vi "Convert Class To Database.vi"(8 "error in (no error)":errorcluster, 10 "table":string, 11 "MemberInfo in":refnum<class "Information.lvclass">) -> (0 "error out":errorcluster, 2 "UserInfo":T1, 3 "MemberInfo out":refnum<class "Information.lvclass">)   [LabVIEW 2015, in "Member_Actor.lvlib" / "Information.lvclass"]
uses:
  Information.lvclass
  Type Definitions/UserInfo.ctl
  Information.lvclass/Information.ctl
  API/_Database/Database.lvclass
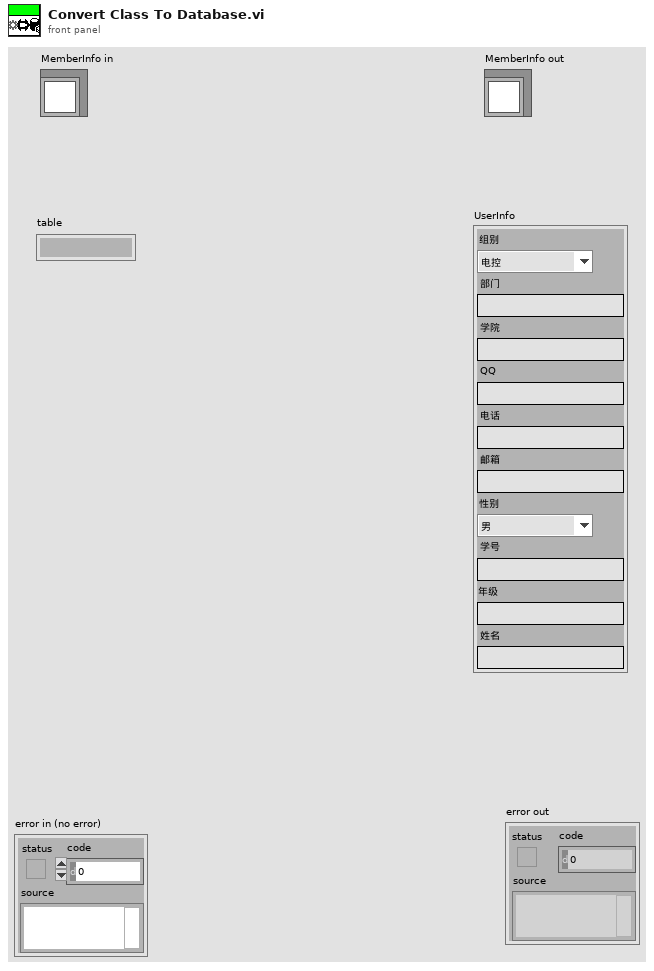
[diagram p1: front panel]
types:
  T1 = typedef "Member_Actor.lvlib/Information.lvclass/UserInfo.ctl" = cluster{"组别":enum16{"电控", "机械", "视觉"}, "部门":string, "学院":string, "QQ":string, "电话":string, "邮箱":string, "性别":enum16{"男", "女"}, "学号":string, "年级":string, "姓名":string}
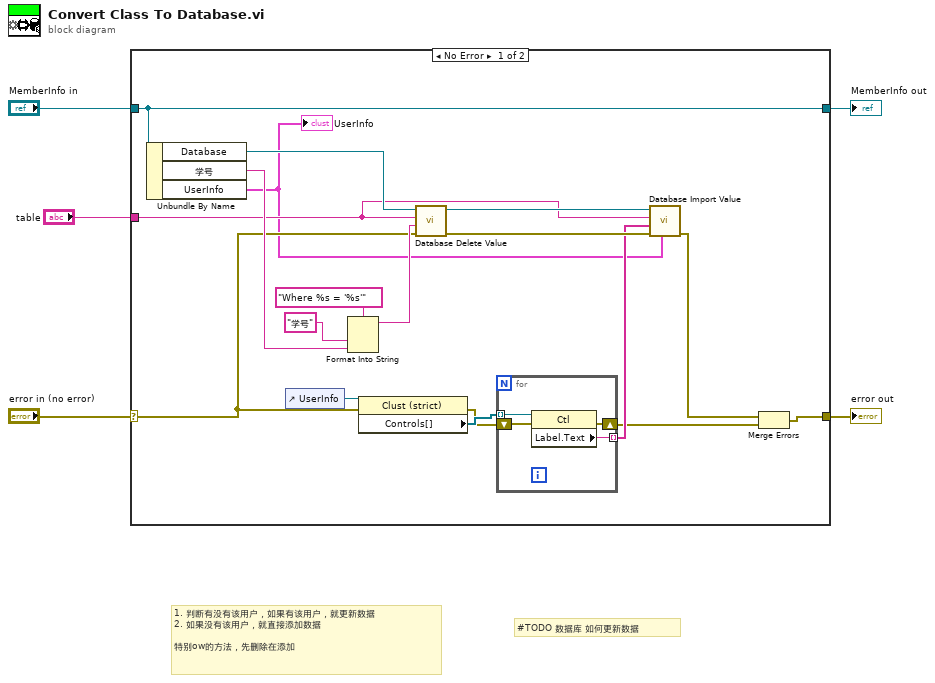
[diagram p0: block diagram]
diagram:
  # "#TODO 数据库 如何更新数据"
  # "1. 判断有没有该用户，如果有该用户，就更新数据\n2. 如果没有该用户，就直接添加数据\n\n特别ow的方法，先删除在添加"
  n1 = case shown="No Error" "error in (no error)" {
    selector: "error in (no error)" -> [w13 w29]
    tunnel: [w6 w29] -> w4
    tunnel: [w23 w28] -> w2
    tunnel: "MemberInfo in" -> [w23 w28]
    tunnel: "table" -> [w15 _]
    frame No Error {
      n2 = Unbundle By Name(w23) -> ("Database"=w22:refnum<class "Database.lvclass">, "学号"=w20:string, "UserInfo"=w9:T1)
      "UserInfo" <- w9
      n3 = control-ref of="UserInfo"() -> (w14:refnum<vi>)
      n4 = Format Into String(format string="Where %s = '%s'", "学号" ("input 1"), w20) -> (resulting string=w18:string)  [unwired: 2 in, 1 out]
      n5 = property class="Clust (strict)"(reference=w14, error in=w13) -> (error out=w11:errorcluster, "Controls[]"=w12:refnum<vi>[])  [unwired: 1 out]
      n6 = call "Database Delete Value.vi"("error in (no error)"=w13, "condition"=w18, "table"=w15, "object in"=w22) -> ("error out"=w16:errorcluster, "object out"=w17:refnum<class "Database.lvclass">)  [unwired: 6 in]
      n7 = for {
        tunnel: w12 -> [w27] mode=indexing
        tunnel: [w25] -> w10 mode=indexing
        shift-right: [w24] -> w7
        shift-left: w11 -> [w26]
        n8 = property class="Ctl"(reference=w27, error in=w26) -> (error out=w24:errorcluster, "Label.Text"=w25:string)  [unwired: 1 out]
      }
      n9 = call "Database Import Value.vi"("data"=w9, "error in (no error)"=w16, "columns"=w10, "table"=w15, "object in"=w17) -> ("error out"=w8:errorcluster)  [unwired: 5 in, 1 out]
      n10 = Merge Errors(w8, w7) -> (w6:errorcluster)
    }
    frame Error {
    }
  }
  "error out" <- w4
  "MemberInfo out" <- w2
